vi "When Write.vi"(0 "error out":errorcluster, 2 "return count":u32, 11 "Serial in":refnum<class "Mock Serial.lvclass">) -> (3 "Serial out":refnum<class "Mock Serial.lvclass">)   [LabVIEW 2020, in "Mock Serial.lvclass"]
uses:
  Mock Serial.lvclass
  Mock Serial.lvclass/Mock Serial.ctl
  <vilib>/Astemes/LMock/Mock.lvclass
  C:/Program Files (x86)/National Instruments/LabVIEW 2020/vi.lib/Astemes/LMock/Mock.lvclass
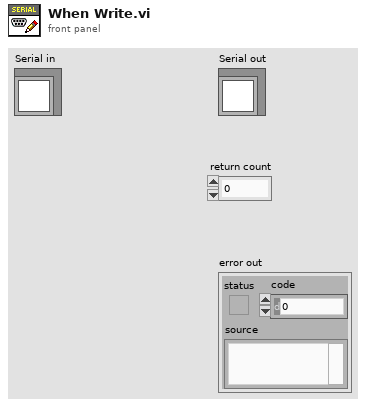
[diagram p1: front panel]
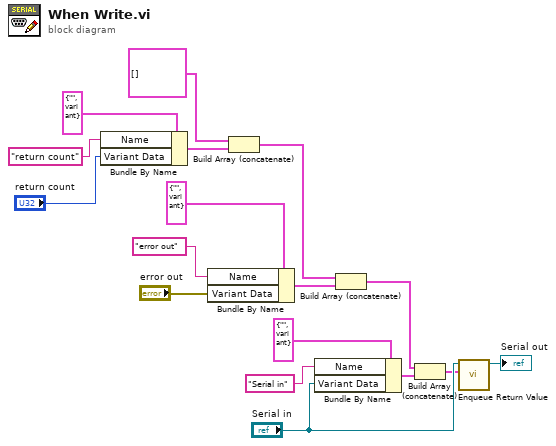
[diagram p0: block diagram]
diagram:
  n1 = Bundle By Name(cluster=cluster{"Name":string, "Variant Data":variant} {"Name"="", "Variant Data"=variant} ("element"), "Name"="return count", "Variant Data"="return count") -> (w5:cluster{"Name":string, "Variant Data":variant})
  n2 = Bundle By Name(cluster=cluster{"Name":string, "Variant Data":variant} {"Name"="", "Variant Data"=variant} ("element"), "Name"="error out", "Variant Data"="error out") -> (w3:cluster{"Name":string, "Variant Data":variant})
  n3 = Build Array (concatenate)(cluster{"Name":string, "Variant Data":variant}[] [] ("Control Values"), w5) -> (w10:cluster{"Name":string, "Variant Data":variant}[])
  n4 = Bundle By Name(cluster=cluster{"Name":string, "Variant Data":variant} {"Name"="", "Variant Data"=variant} ("element"), "Name"="Serial in", "Variant Data"="Serial in") -> (w1:cluster{"Name":string, "Variant Data":variant})
  n5 = Build Array (concatenate)(w10, w3) -> (w13:cluster{"Name":string, "Variant Data":variant}[])
  n6 = Build Array (concatenate)(w13, w1) -> (w15:cluster{"Name":string, "Variant Data":variant}[])
  n7 = call <vilib>:"Enqueue Return Value.vi"("Indicator Values"=w15, "Mock In"="Serial in") -> ("Mock Out"=→"Serial out":refnum<class "Mock Serial.lvclass">)  [unwired: 8 in, 1 out]
